vi "run_fgv.vi"(7 "mode":enum16{"read", "write"}(ring), 9 "passed":bool, 10 "error in (no error)":errorcluster, 11 "date in":T1) -> (1 "passed":bool, 2 "error out":errorcluster, 3 "date 0ut":T1)   [LabVIEW 2019]
uses:
  core_autoMonitorDataCluster.ctl
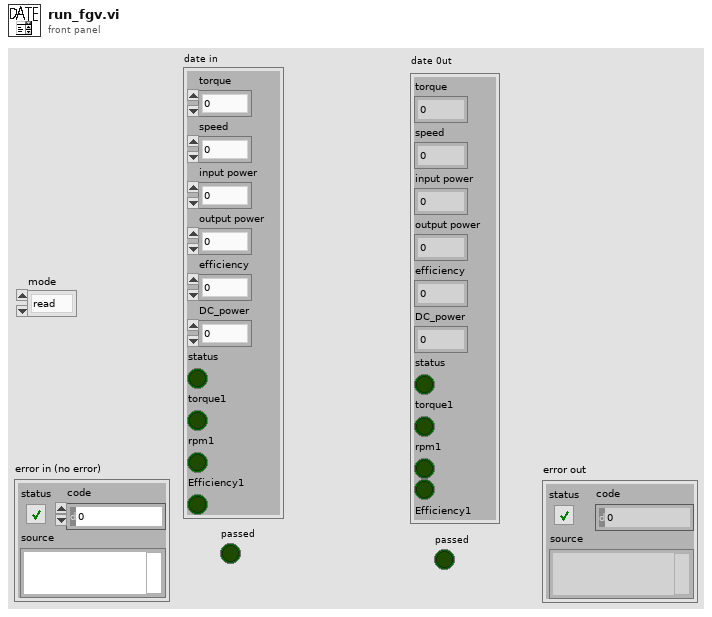
[diagram p1: front panel]
types:
  T1 = typedef "core_autoMonitorDataCluster.ctl" = cluster{"torque":dbl, "speed":dbl, "input power":dbl, "output power":dbl, "efficiency":dbl, "DC_power":dbl, "status":bool, "torque1":bool, "rpm1":bool, "Efficiency1":bool}
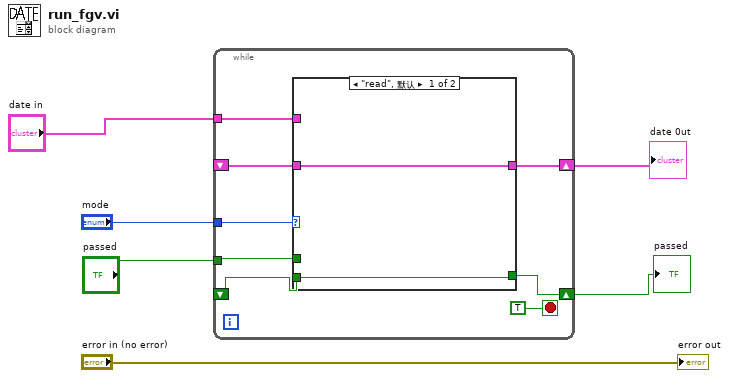
[diagram p0: block diagram]
diagram:
  n1 = while {
    tunnel: "mode" -> [w14]
    tunnel: "date in" -> [w13]
    shift-right: [w12] -> w3
    shift-left: _ -> [w11]
    shift-right: [w9] -> w2
    shift-left: _ -> [w8]
    tunnel: "passed" -> [w7]
    stop <- TRUE stop-if-true
    n2 = case shown="\"read\", 默认" w14 {
      tunnel: [w16 w18] -> w12
      tunnel: w13 -> [_ w18]
      tunnel: w11 -> [w16 _]
      tunnel: [w15 w17] -> w9
      tunnel: w8 -> [w15 _]
      tunnel: w7 -> [_ w17]
      frame "read", Default {
      }
      frame "write" {
      }
    }
  }
  "date 0ut" <- w3
  "passed" <- w2
  "error out" <- "error in (no error)"
